vi "GetPoupMenus.vi"(11 "Configurations":string[](array[string])) -> (1 "PopUpMenu(IfExists)":T1[](array[typedef]))   [LabVIEW 2020, in "DependencyViewer.lvlib"]
uses:
  DependencyViewer.lvlib
  <resource>/Framework/Providers/API/mxLvMenuItem.ctl
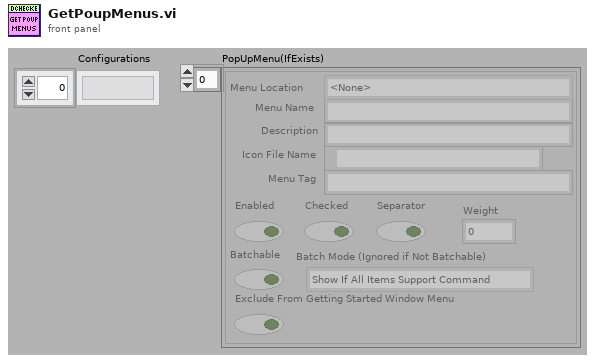
[diagram p1: front panel]
types:
  T1 = typedef "mxLvMenuItem.ctl" = cluster{"Menu Name":string, "Description":string, "Icon File Name":path, "Menu Tag":string, "Enabled":bool, "Checked":bool, "Separator":bool, "Batchable":bool, "Weight":i32, "Batch Mode (Ignored if Not Batchable)":enum32{"Show If All Items Support Command", "Show If Any Items Support Command"}, "Menu Location":enum32{"<None>", "Project", "Project / Build Specifications", "Tools", "Tools / Source Control", "Tools / Real-Time Module", "Help"}, "Exclude From Getting Started Window Menu":bool}
  T2 = typedef "DependencyViewer.lvlib/Settings.ctl" = cluster{"EmbedChartLibraryScript":bool, "Configurations":T3[], "UseProjectFolder":bool, "Folder to save reports to":path, "Max reports to save":u8}
  T3 = typedef "DependencyViewer.lvlib/DependencyConfiguration.ctl" = cluster{"Name":string, "RemoveItemsBelongingToLibraries":bool, "RemoveEvenSubLibraries":bool, "FilterOptions":T4, "OnlyKeepCircularDepedencies":bool, "IgnoreLibrariesInCircularDependencies":bool}
  T4 = typedef "DependencyViewer.lvlib/FilterOptions.ctl" = cluster{"Ignore user.lib":bool, "Ignore vi.lib":bool, "Ignore instr.lib":bool, "FolderToIgnore":path[], "Ignore libraries":bool, "Ignore lvcasses":bool, "Ignore xnodes":bool, "Ignore xcontrols":bool, "Ignore Channel Classes":bool}
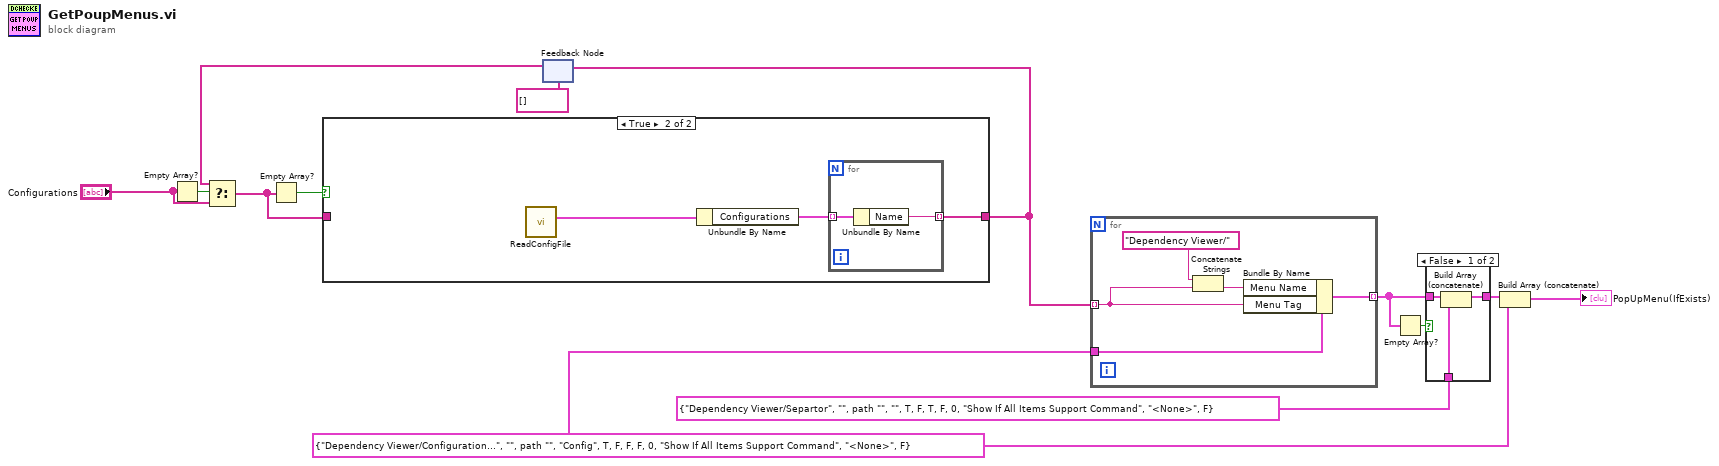
[diagram p0: block diagram]
diagram:
  w1 = T1 {"Menu Name"="Dependency Viewer/Configuration...", "Description"="", "Icon File Name"=path "", "Menu Tag"="Config", "Enabled"=TRUE, "Checked"=FALSE, "Separator"=FALSE, "Batchable"=FALSE, "Weight"=0, "Batch Mode (Ignored if Not Batchable)"=enum."Show If All Items Support Command", "Menu Location"=enum."<None>", "Exclude From Getting Started Window Menu"=FALSE} ("Menu Item")
  n1 = Empty Array?(array="Configurations") -> (empty?=w10:bool)
  n2 = feedback #1(string[] [] ("Configurations")) -> (w9:string[])
  n3 = Select(t=w9, s=w10, f="Configurations") -> (s? t:f=w7:string[])
  n4 = Empty Array?(array=w7) -> (empty?=w8:bool)
  n5 = case shown="True" w8 {
    tunnel: [w14 w16] -> w6
    tunnel: w7 -> [w14 _]
    frame False {
    }
    frame True {
      n6 = call "ReadConfigFile.vi"() -> ("Config"=w15:T2)  [unwired: 11 in]
      n7 = Unbundle By Name(w15) -> ("Configurations"=w17:T3[])
      n8 = for {
        tunnel: w17 -> [w19] mode=indexing
        tunnel: [w18] -> w16 mode=indexing
        n9 = Unbundle By Name(w19) -> ("Name"=w18:string)
      }
    }
  }
  n10 = feedback-in #1(w6) -> ()
  n11 = for {
    tunnel: w1 -> [w24]
    tunnel: w6 -> [w20] mode=indexing
    tunnel: [w21] -> w5 mode=indexing
    n12 = Concatenate Strings("Dependency Viewer/" ("string"), w20) -> (w23:string)
    n13 = Bundle By Name(cluster=w24, "Menu Name"=w23, "Menu Tag"=w20) -> (w21:T1)
  }
  n14 = Empty Array?(array=w5) -> (empty?=w4:bool)
  n15 = case shown="False" w4 {
    tunnel: w5 -> [w27 w28]
    tunnel: T1 {"Menu Name"="Dependency Viewer/Separtor", "Description"="", "Icon File Name"=path "", "Menu Tag"="", "Enabled"=TRUE, "Checked"=FALSE, "Separator"=TRUE, "Batchable"=FALSE, "Weight"=0, "Batch Mode (Ignored if Not Batchable)"=enum."Show If All Items Support Command", "Menu Location"=enum."<None>", "Exclude From Getting Started Window Menu"=FALSE} ("Menu Item") -> [w26 _]
    tunnel: [w25 w28] -> w2
    frame False {
      n16 = Build Array (concatenate)(w27, w26) -> (w25:T1[])
    }
    frame True {
    }
  }
  n17 = Build Array (concatenate)(w2, w1) -> (→"PopUpMenu(IfExists)":T1[])
